vi "Resolve Redirects.vi"(6 "timeout (10000)":i32=10000, 7 "max redirects":i32=21, 8 "error in (no error)":errorcluster, 11 "URL":string) -> (0 "error out":errorcluster, 3 "URL out":string)   [LabVIEW 2020, in "binary_installation_tools.lvlib"]
uses:
  binary_installation_tools.lvlib
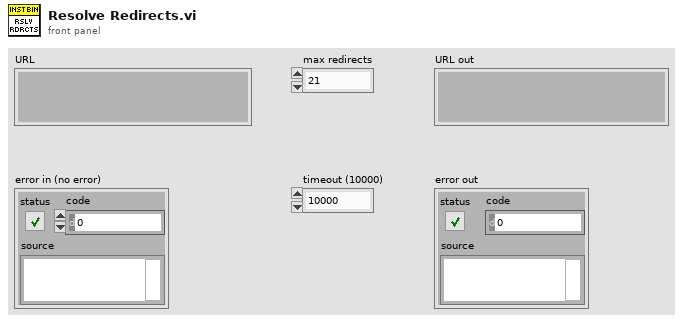
[diagram p1: front panel]
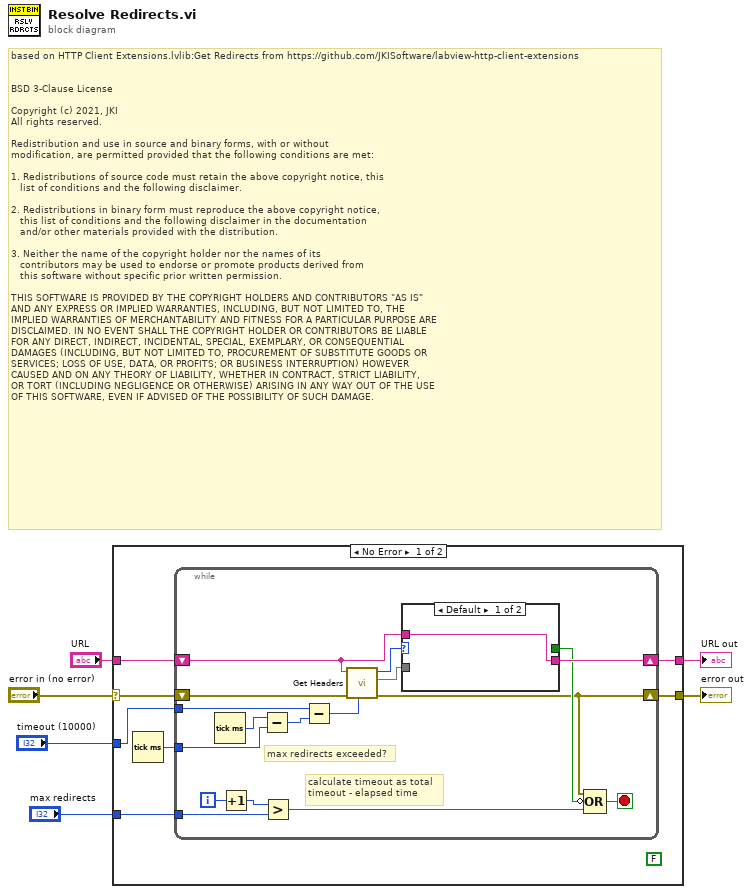
[diagram p0: block diagram]
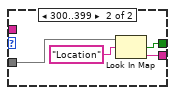
[diagram p2: hidden frame]
diagram:
  # "based on HTTP Client Extensions.lvlib:Get Redirects from https://github.com/JKISoftware/labview-http-client-extensions\n\n\nBSD 3-Clause License\n\nCopyright (c) 2021, JKI\nAll rights reserved.\n\nRedistribution and use in source and binary forms, with or without\nmodification, are permitted provided that the following conditions are met:\n\n1. Redistributions of source code must retain the above copyright notice, this\n   list of conditions and the following disclaimer.\n\n2. Redistributions in binary form must reproduce the above copyright notice,\n   this list of conditions and the following disclaimer in the documentation\n   and/or other materials provided with the distribution.\n\n3. Neither the name of the copyright holder nor the names of its\n   contributors may be used to endorse or promote products derived from\n   this software without specific prior written permission.\n\nTHIS SOFTWARE IS PROVIDED BY THE COPYRIGHT HOLDERS AND CONTRIBUTORS \"AS IS\"\nAND ANY EXPRESS OR IMPLIED WARRANTIES, INCLUDING, BUT NOT LIMITED TO, THE\nIMPLIED WARRANTIES OF MERCHANTABILITY AND FITNESS FOR A PARTICULAR PURPOSE ARE\nDISCLAIMED. IN NO EVENT SHALL THE COPYRIGHT HOLDER OR CONTRIBUTORS BE LIABLE\nFOR ANY DIRECT, INDIRECT, INCIDENTAL, SPECIAL, EXEMPLARY, OR CONSEQUENTIAL\nDAMAGES (INCLUDING, BUT NOT LIMITED TO, PROCUREMENT OF SUBSTITUTE GOODS OR\nSERVICES; LOSS OF USE, DATA, OR PROFITS; OR BUSINESS INTERRUPTION) HOWEVER\nCAUSED AND ON ANY THEORY OF LIABILITY, WHETHER IN CONTRACT, STRICT LIABILITY,\nOR TORT (INCLUDING NEGLIGENCE OR OTHERWISE) ARISING IN ANY WAY OUT OF THE USE\nOF THIS SOFTWARE, EVEN IF ADVISED OF THE POSSIBILITY OF SUCH DAMAGE."
  n1 = case shown="No Error" "error in (no error)" {
    selector: "error in (no error)" -> [w11 w36]
    tunnel: "URL" -> [w13 w37]
    tunnel: [w12 w36] -> w5
    tunnel: [w10 w37] -> w3
    tunnel: "max redirects" -> [w9 _]
    tunnel: "timeout (10000)" -> [w8 _]
    frame No Error {
      (unwired) FALSE
      n2 = Tick Count (ms)() -> (millisecond timer value=w7:u32)
      n3 = while {
        shift-right: [w29] -> w10
        shift-left: w13 -> [w15]
        shift-right: [w18] -> w12
        shift-left: w11 -> [w19]
        tunnel: w9 -> [w27]
        tunnel: w8 -> [w22]
        tunnel: w7 -> [w24]
        i -> [w20]
        stop <- w30 stop-if-true
        # "max redirects exceeded?"
        # "calculate timeout as total timeout - elapsed time"
        n4 = Tick Count (ms)() -> (millisecond timer value=w25:u32)
        n5 = Increment(x=w20) -> (x+1=w21:i32)
        n6 = Subtract(x=w25, y=w24) -> (x-y=w23:u32)
        n7 = Greater?(x=w21, y=w27) -> (0:w26:bool)
        n8 = Subtract(x=w22, y=w23) -> (x-y=w14:u32)
        n9 = call "Get Headers.vi"("timeout (10000)"=w14, "error in (no error)"=w19, "URL"=w15) -> ("error out"=w18:errorcluster, "Headers"=w16:map{string, string}, "Reponse Code"=w17:i32)  [unwired: 3 in, 3 out]
        n10 = case shown="Default" w17 {
          tunnel: [w31 w33] -> w29
          tunnel: [_ w32] -> w28
          tunnel: w15 -> [w31 _]
          tunnel: w16 -> [_ w35]
          frame Default {
          }
          frame 300..399 {
            n11 = Look In Map(map=w35, key="Location" ("header")) -> (key not found?=w32:bool, value=w33:string)  [unwired: 1 in]
          }
        }
        n12 = Compound Arithmetic op=OR(w18, invert w28, w26) -> (w30:bool)
      }
    }
    frame Error {
    }
  }
  "URL out" <- w3
  "error out" <- w5
